vi "TestData_Initial.vi"(7 "Close Connect?":bool, 8 "error in (no error)":errorcluster caption="错误输入（无错误）", 9 "Root Path":path=path "d:/", 10 "Tables_Exist?":string, 11 "ConnectionString":T1={"IP"="localhost", "Port"="3306", "DataBase"="uel_te", "User"="root", "Password"="alpha130723"}) -> (0 "error out":errorcluster, 1 "Report path":path=path "d:/reports", 2 "ADODB._Connection Out":refnum<k7>, 3 "Status":cluster{"DataBase":bool, "NetDisk":bool}={"DataBase"=TRUE, "NetDisk"=TRUE})   [LabVIEW 2012, in "Lib_UEL.ATE.lvlib" / "Lib_TestData.lvlib"]
uses:
  Lib_TestData.lvlib
  <vilib>/regexp/Match Regular Expression.xnode
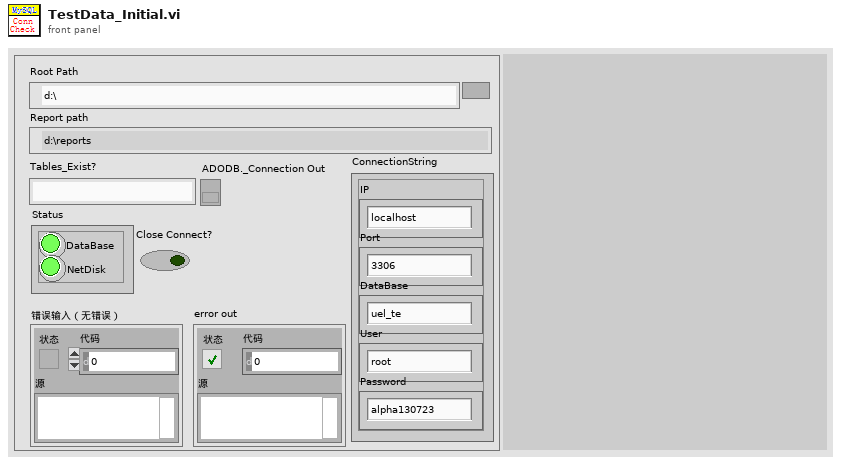
[diagram p1: front panel]
types:
  T1 = cluster{"IP":string, "Port":string, "DataBase":string, "User":string, "Password":string}
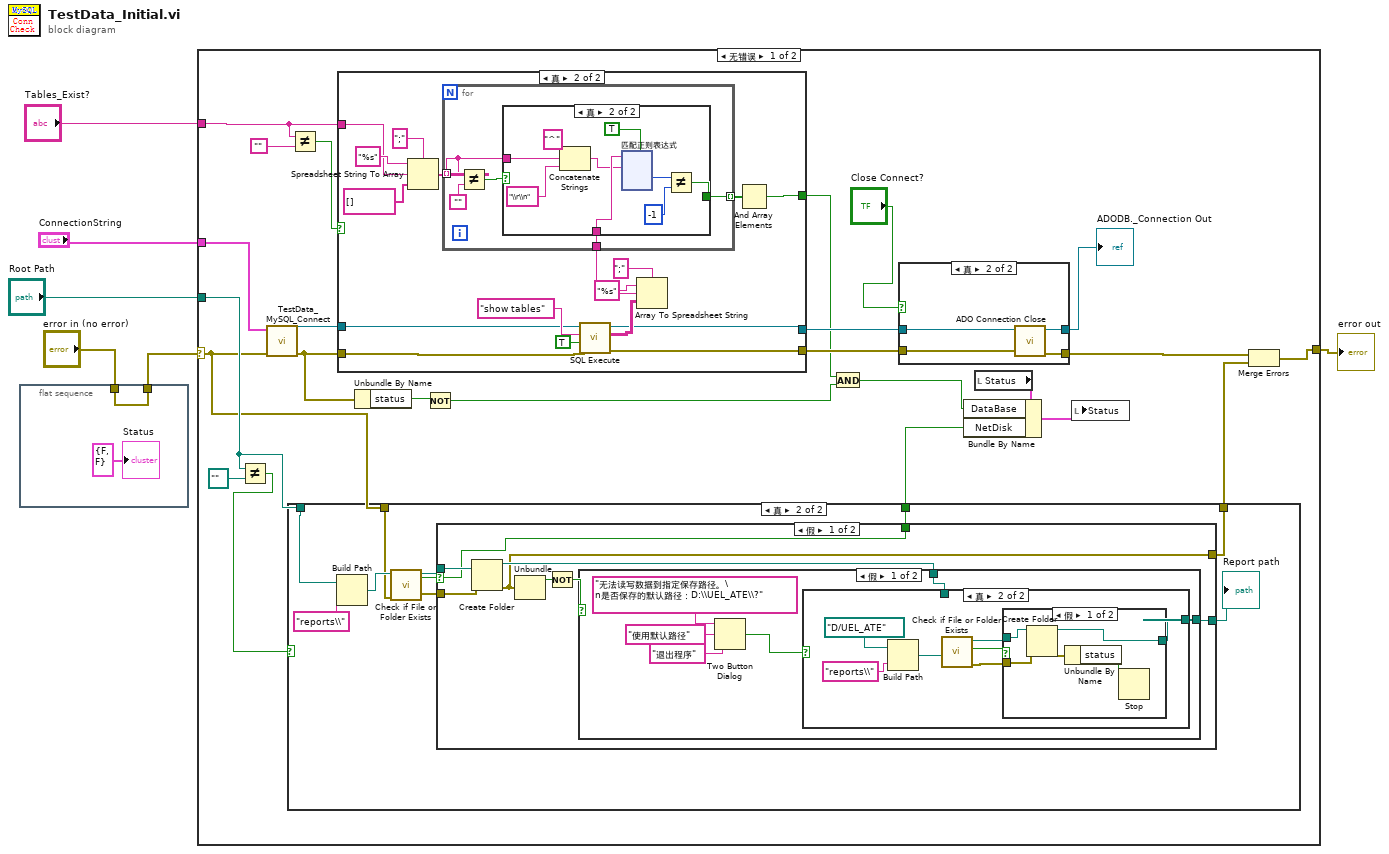
[diagram p0: block diagram]
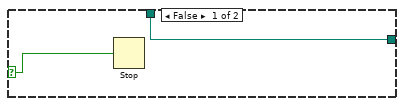
[diagram p4: hidden frame]
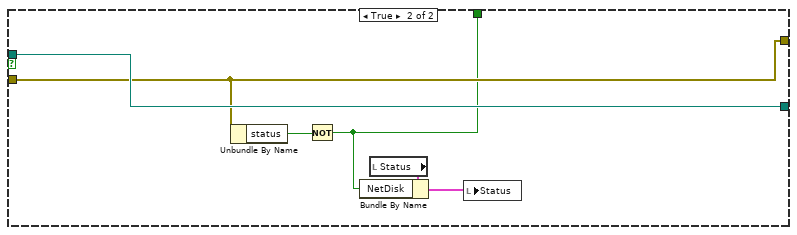
[diagram p7: hidden frame]
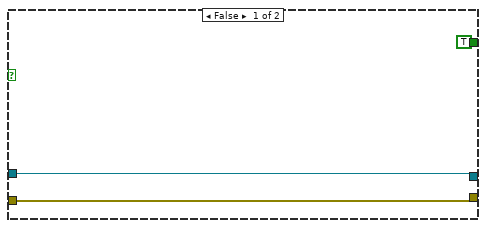
[diagram p8: hidden frame]
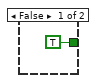
[diagram p9: hidden frame]
diagram:
  n1 = flat-sequence {
    tunnel: [w8] -> w5
    tunnel: "error in (no error)" -> [w8]
    frame #0 {
      "Status" <- cluster{"DataBase":bool, "NetDisk":bool} {"DataBase"=FALSE, "NetDisk"=FALSE} ("Status")
    }
  }
  n2 = case shown="无错误" w5 {
    selector: w5 -> [w15 w233]
    tunnel: [w11 w233] -> w6
    tunnel: "ConnectionString" -> [w32 _]
    tunnel: "Tables_Exist?" -> [w31 _]
    tunnel: "Root Path" -> [w16 _]
    frame No Error {
      n3 = Not Equal?(x=w16, y=path "") -> (x != y?=w17:bool)
      n4 = call "TestData_MySQL_Connect.vi"("error in (no error)"=w15, "ConnectionString"=w32) -> ("Error Out"=w27:errorcluster, "Connection Out"=w28:refnum<k7>)  [unwired: 8 in]
      n5 = case shown="真" w17 {
        selector: w17 -> [w40 _]
        tunnel: w16 -> [_ w44]
        tunnel: w15 -> [w39 w43]
        tunnel: [w40 w42] -> w14
        tunnel: [w39 w41] -> w13
        frame False {
        }
        frame True {
          n6 = Build Path(base path=w44, name or relative path="reports\\" ("名称或相对路径")) -> (appended path=w46:path)
          n7 = call <vilib>:"Check if File or Folder Exists.vi"("error in (no error)"=w43, "path"=w46) -> ("error out"=w47:errorcluster, "file or folder exists?"=w49:bool, "dup path"=w48:path)  [unwired: 7 in]
          n8 = case shown="假" w49 {
            selector: w49 -> [w51 _]
            tunnel: [w54 w86] -> w45
            tunnel: w48 -> [w57 w86]
            tunnel: w47 -> [w58 w85]
            tunnel: [w52 w85] -> w41
            tunnel: [w51 w81] -> w42
            frame False {
              n9 = Create Folder(path (use dialog)=w57, error in=w58) -> (created path=w53:path, error out=w52:errorcluster)  [unwired: 1 in, 1 out]
              n10 = Unbundle(w52) -> ("status"=w56:bool)  [unwired: 2 out]
              n11 = Not(x=w56) -> (.not. x?=w55:bool)
              n12 = case shown="假" w55 {
                tunnel: [w63 w80] -> w54
                tunnel: w53 -> [w62 w80]
                frame False {
                  n13 = Two Button Dialog(message="无法读写数据到指定保存路径。\n是否保存的默认路径：D:\\UEL_ATE\\?" ("消息"), 1:"退出程序" ("F按钮名称（“取消”）"), 2:"使用默认路径" ("T按钮名称（“确定”）")) -> (T button?=w61:bool)
                  n14 = case shown="真" w61 {
                    selector: w61 -> [w65 _]
                    tunnel: [w66 w67] -> w63
                    tunnel: w62 -> [w66 _]
                    frame False {
                      n15 = Stop(stop? (T)=w65) -> ()
                    }
                    frame True {
                      n16 = Build Path(base path=path "D:/UEL_ATE" ("基路径"), name or relative path="reports\\" ("名称或相对路径")) -> (appended path=w71:path)
                      n17 = call <vilib>:"Check if File or Folder Exists.vi"("path"=w71) -> ("error out"=w69:errorcluster, "file or folder exists?"=w68:bool, "dup path"=w70:path)  [unwired: 8 in]
                      n18 = case shown="假" w68 {
                        tunnel: w70 -> [w76 w79]
                        tunnel: [w78 w79] -> w67
                        tunnel: w69 -> [w77 _]
                        frame False {
                          n19 = Create Folder(path (use dialog)=w76, error in=w77) -> (created path=w78:path, error out=w75:errorcluster)  [unwired: 1 in, 1 out]
                          n20 = Unbundle By Name(w75) -> ("status"=w74:bool)
                          n21 = Stop(stop? (T)=w74) -> ()
                        }
                        frame True {
                        }
                      }
                    }
                  }
                }
                frame True {
                }
              }
            }
            frame True {
              n22 = Unbundle By Name(w85) -> ("status"=w84:bool)
              n23 = Not(x=w84) -> (.not. x?=w81:bool)
              n24 = local read "Status"() -> (w83:cluster{"DataBase":bool, "NetDisk":bool})
              n25 = Bundle By Name(cluster=w83, "NetDisk"=w81) -> (w82:cluster{"DataBase":bool, "NetDisk":bool})
              n26 = local write "Status"(w82) -> ()
            }
          }
          "Report path" <- w45
        }
      }
      n27 = Not Equal?(x=w31, y="") -> (x != y?=w22:bool)
      n28 = case shown="真" w22 {
        tunnel: [w88 w106] -> w30
        tunnel: [w89 w90] -> w29
        tunnel: w28 -> [w89 w91]
        tunnel: w27 -> [w88 w105]
        tunnel: [TRUE w94] -> w25
        tunnel: w31 -> [_ w93]
        frame False {
        }
        frame True {
          n29 = Spreadsheet String To Array(delimiter (Tab)=";" ("分隔符(Tab)"), format string="%s" ("格式字符串"), spreadsheet string=w93, array type (2D Dbl)=string[] []) -> (array=w96:string[])
          n30 = call <userlib>:"SQL Execute.vi"("error in (no error)"=w105, "Return Data (T)"=TRUE, "Command Text"="show tables", "ADODB._Connection In"=w91) -> ("error out"=w106:errorcluster, "Data"=w99:string[][], "ADODB._Connection Out"=w90:refnum<k7>)  [unwired: 4 in, 1 out]
          n31 = Array To Spreadsheet String(delimiter (Tab)=";" ("分隔符(Tab)"), array=w99, 3:"%s" ("格式字符串")) -> (spreadsheet string=w92:string)
          n32 = for {
            tunnel: w96 -> [w109] mode=indexing
            tunnel: w92 -> [w110]
            tunnel: [w111] -> w95 mode=indexing
            n33 = Not Equal?(x=w109, y="") -> (x != y?=w107:bool)
            n34 = case shown="真" w107 {
              tunnel: [TRUE w120] -> w111
              tunnel: w110 -> [_ w119]
              tunnel: w109 -> [_ w116]
              frame False {
              }
              frame True {
                n35 = Concatenate Strings("^" ("字符串"), w116, "\\r\\n" ("字符串")) -> (w115:string)
                n36 = xnode "匹配正则表达式"("输入字符串"=w119, "正则表达式"=w115, "多行？(F)"=TRUE) -> ("匹配后偏移量"=w118:i32)  [unwired: 3 in, 4 out]
                n37 = Not Equal?(x=w118, y=-1) -> (x != y?=w120:bool)
              }
            }
          }
          n38 = And Array Elements(Boolean array=w95) -> (logical AND=w94:bool)
        }
      }
      n39 = Unbundle By Name(w27) -> ("status"=w26:bool)
      n40 = Not(x=w26) -> (.not. x?=w24:bool)
      n41 = And(x=w25, y=w24) -> (x .and. y?=w19:bool)
      n42 = case shown="真" "Close Connect?" {
        tunnel: w30 -> [w33 w38]
        tunnel: w29 -> [w34 w37]
        tunnel: [w33 w36] -> w12
        tunnel: [w34 w35] -> w9
        frame False {
        }
        frame True {
          n43 = call <userlib>:"ADO Connection Close.vi"("error in (no error)"=w38, "ADODB._Connection In"=w37) -> ("error out"=w36:errorcluster, "ADODB._Connection Out"=w35:refnum<k7>)  [unwired: 8 in]
        }
      }
      "ADODB._Connection Out" <- w9
      n44 = local read "Status"() -> (w21:cluster{"DataBase":bool, "NetDisk":bool})
      n45 = Bundle By Name(cluster=w21, "DataBase"=w19, "NetDisk"=w14) -> (w20:cluster{"DataBase":bool, "NetDisk":bool})
      n46 = local write "Status"(w20) -> ()
      n47 = Merge Errors(w12, w13) -> (w11:errorcluster)
    }
    frame Error {
    }
  }
  "error out" <- w6
